vi "UICtrls_Read_Name.vi"() -> ()   [LabVIEW 2025]
uses:
  UI_Manager.lvlib
panel:
  out "Data":variant
  out "Message":string
  out "Reply Queue":refnum<queue>
  in  "Control Value":variant
  in  "Control Label":string
  out "error out":errorcluster
  in  "error in":errorcluster
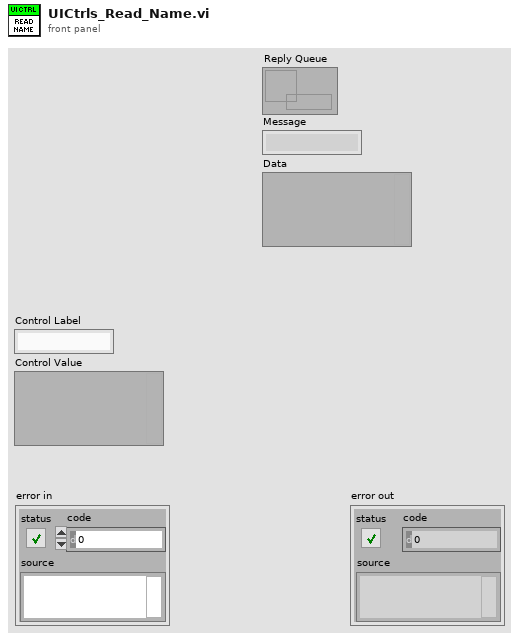
[diagram p1: front panel]
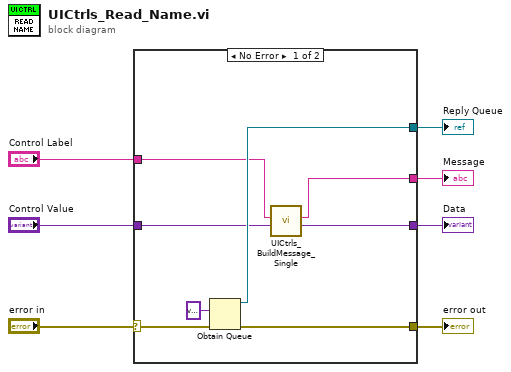
[diagram p0: block diagram]
diagram:
  n1 = case shown="No Error" "error in" {
    selector: "error in" -> [w14 w16]
    tunnel: "Control Value" -> [w11 _]
    tunnel: "Control Label" -> [w10 _]
    tunnel: [w13 _] -> w4
    tunnel: [w12 w16] -> w3
    tunnel: [w9 _] -> w2
    tunnel: [w8 _] -> w1
    frame No Error {
      n2 = Obtain Queue(element data type=variant, error in (no error)=w14) -> (queue out=w13:refnum<queue>, error out=w12:errorcluster)  [unwired: 3 in, 1 out]
      n3 = call "UICtrls_BuildMessage_Single.vi"("Control Label"=w10, "Control Data"=w11) -> ("Message"=w9:string, "Data"=w8:variant)  [unwired: 5 in]
    }
    frame Error {
    }
  }
  "error out" <- w3
  "Reply Queue" <- w4
  "Message" <- w2
  "Data" <- w1
